vi "Color_Textbox.vi"(3 "TypeResult":u8, 5 "Text":string) -> (1 "01":string)   [LabVIEW 2017]
panel:
  # "Type Resule\n0 = Stand by\n1 = OK\n5 = NG"
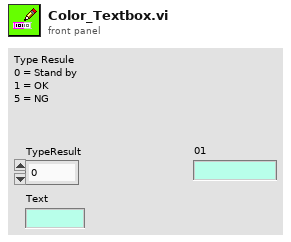
[diagram p1: front panel]
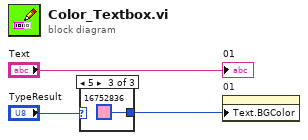
[diagram p0: block diagram]
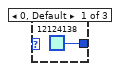
[diagram p2: hidden frame]
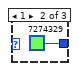
[diagram p3: hidden frame]
diagram:
  n1 = case shown="5" "TypeResult" {
    tunnel: [u32 12124138 u32 7274329 u32 16752836] -> w2
    frame 0, Default {
    }
    frame 1 {
    }
    frame 5 {
    }
  }
  n2 = property on="01" class="Str"("Text.BGColor"=w2) -> ()  [unwired: 2 in, 2 out]
  "01" <- "Text"
